vi "human_interface_2w_with2rows.vi"() -> ()   [LabVIEW 2023]
uses:
  <vilib>/MakerHub/LINX/Public/Peripherals/Digital/Digital Read 1 Chan.vi
  <vilib>/MakerHub/LINX/Public/Peripherals/Digital/Digital Write 1 Chan.vi
  <vilib>/MakerHub/LINX/Public/Peripherals/Digital/Digital Read N Chans.vi
  <vilib>/MakerHub/LINX/Public/Peripherals/Digital/Digital Write N Chans.vi
  <vilib>/MakerHub/LINX/Private/Local IO/LinxDigitalRead.vi
  <vilib>/MakerHub/LINX/Public/Utilities/Check Channel.vi
  <vilib>/MakerHub/LINX/Private/Local IO/LinxDigitalWrite.vi
  <vilib>/MakerHub/LINX/Public/Utilities/Open Serial.vi
  <vilib>/MakerHub/LINX/Private/Utilties/Generate Error.vi
  <vilib>/MakerHub/LINX/LMH-LINX.lvlib
panel:
  in  "stop":bool
  in  "DO Channel":u8=3
  in  "DI Channel":u8=2
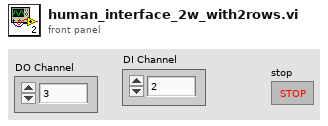
[diagram p1: front panel]
types:
  T1 = typedef "LMH-LINX.lvlib/LINX Ref.ctl" = cluster{"IO":T2, "Interface":T3, "LINX Device Config":T4}
  T2 = typedef "LMH-LINX.lvlib/Platform.ctl" = enum16{"Remote", "Local"}
  T3 = typedef "LMH-LINX.lvlib/Interface.ctl" = enum16{"Serial", "TCP"}
  T4 = typedef "LMH-LINX.lvlib/Device.lvlib/LINX Device Config.ctl" = cluster{"Interface":T3, "COM Port":refnum<visa-resource-name>, "TCP Configuration":T5, "Device Family":u8, "Device ID":u8, "Device Name":string, "TCP Ref":refnum<k5>, "Channels":T6}
  T5 = typedef "LMH-LINX.lvlib/Device.lvlib/TCP Config.ctl" = cluster{"IP Address":string, "Port":u16}
  T6 = typedef "LMH-LINX.lvlib/Channels.ctl" = cluster{"DI":u8[], "DO":u8[], "AI":u8[], "AO":u8[], "PWM":u8[], "QE":u8[], "UART":u8[], "I2C 2":u8[], "SPI":u8[], "CAN":u8[], "Servo":u8[], "AI Ref (V)":dbl, "AI Resolution (Bits)":u8, "AO Ref (V)":dbl, "AO Resolution (Bits)":u8}
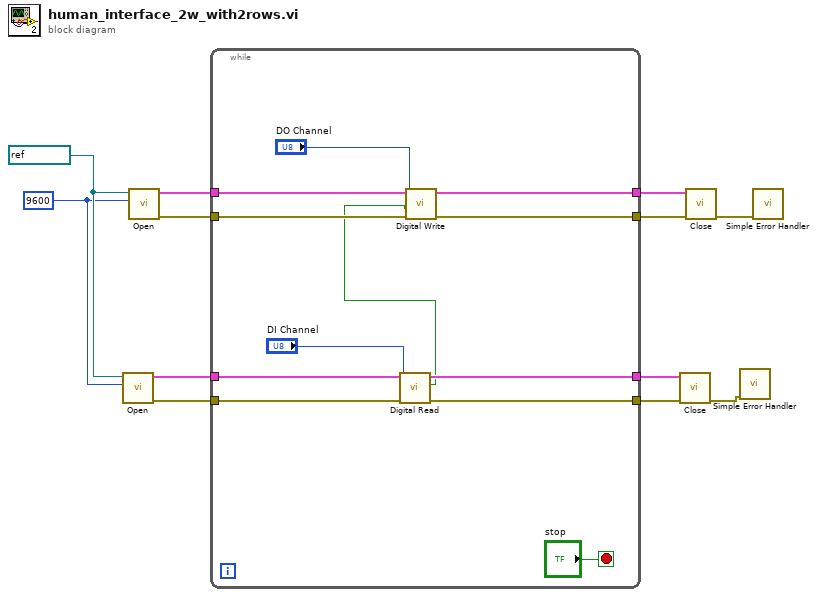
[diagram p0: block diagram]
diagram:
  w2 = u32 9600 ("Baud Rate Override")
  w3 = refnum<visa-resource-name> "COM7" ("Serial Port")
  n1 = call-poly <vilib>:"Open.vi"("Baud Rate Override"=w2, "Serial Port"=w3) -> ("Error Out"=w6:errorcluster, "LINX Resource"=w4:T1)  [unwired: 7 in, 1 out]
  n2 = call-poly <vilib>:"Open.vi"("Baud Rate Override"=w2, "Serial Port"=w3) -> ("Error Out"=w10:errorcluster, "LINX Resource"=w12:T1)  [unwired: 7 in, 1 out]
  n3 = while {
    tunnel: w12 -> [w24]
    tunnel: [w23] -> w11
    tunnel: w10 -> [w22]
    tunnel: [w21] -> w9
    tunnel: w4 -> [w17]
    tunnel: [w18] -> w5
    tunnel: w6 -> [w19]
    tunnel: [w20] -> w7
    stop <- "stop" stop-if-true
    n4 = call-poly <vilib>:"Digital Read.vi"("Error In"=w19, "DI Channel"="DI Channel", "LINX Resource"=w17) -> ("Error Out"=w20:errorcluster, "DI Value"=w14:bool, "LINX Resource"=w18:T1)  [unwired: 6 in]
    n5 = call-poly <vilib>:"Digital Write.vi"("Error In"=w22, "Output Value"=w14, "DO Channel"="DO Channel", "LINX Resource"=w24) -> ("Error Out"=w21:errorcluster, "LINX Resource"=w23:T1)  [unwired: 6 in]
  }
  n6 = call <vilib>:"Close.vi"("Error In"=w7, "LINX Resource"=w5) -> ("Error Out"=w1:errorcluster)  [unwired: 9 in]
  n7 = call <vilib>:"Close.vi"("Error In"=w9, "LINX Resource"=w11) -> ("Error Out"=w8:errorcluster)  [unwired: 9 in]
  n8 = call <vilib>:"Simple Error Handler.vi"("error in (no error)"=w1) -> ()  [unwired: 4 in, 5 out]
  n9 = call <vilib>:"Simple Error Handler.vi"("error in (no error)"=w8) -> ()  [unwired: 4 in, 5 out]
